vi "Get Algorithms.vi"(6 "Backend engine":T1, 8 "error in":errorcluster) -> (0 "error out":errorcluster, 3 "Available Algorithms":T2[](array[typedef]))   [LabVIEW 2013]
doc: "Get informations on all available Algorithms."
uses:
  TD Algorithm Information.ctl
  TD Backend Engine.ctl
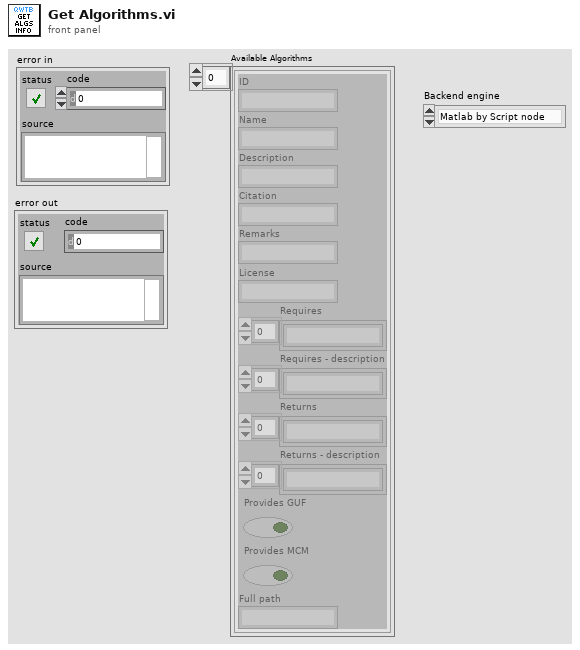
[diagram p1: front panel]
types:
  T1 = typedef "TD Backend Engine.ctl" = enum16{"Matlab by Script node", "GNU Octave by GOLPI"}
  T2 = typedef "TD Algorithm Information.ctl" = cluster{"ID":string, "Name":string, "Description":string, "Citation":string, "Remarks":string, "License":string, "Requires":string[], "Requires - description":string[], "Returns":string[], "Returns - description":string[], "Provides GUF":bool, "Provides MCM":bool, "Full path":string}
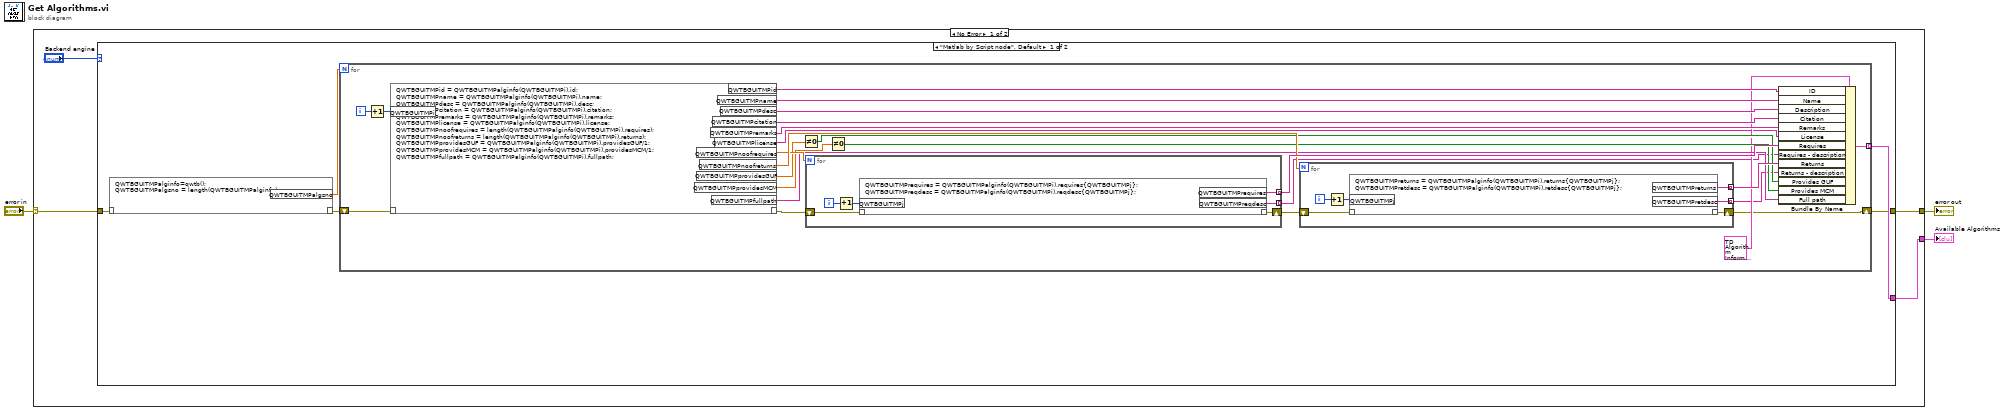
[diagram p0: block diagram]
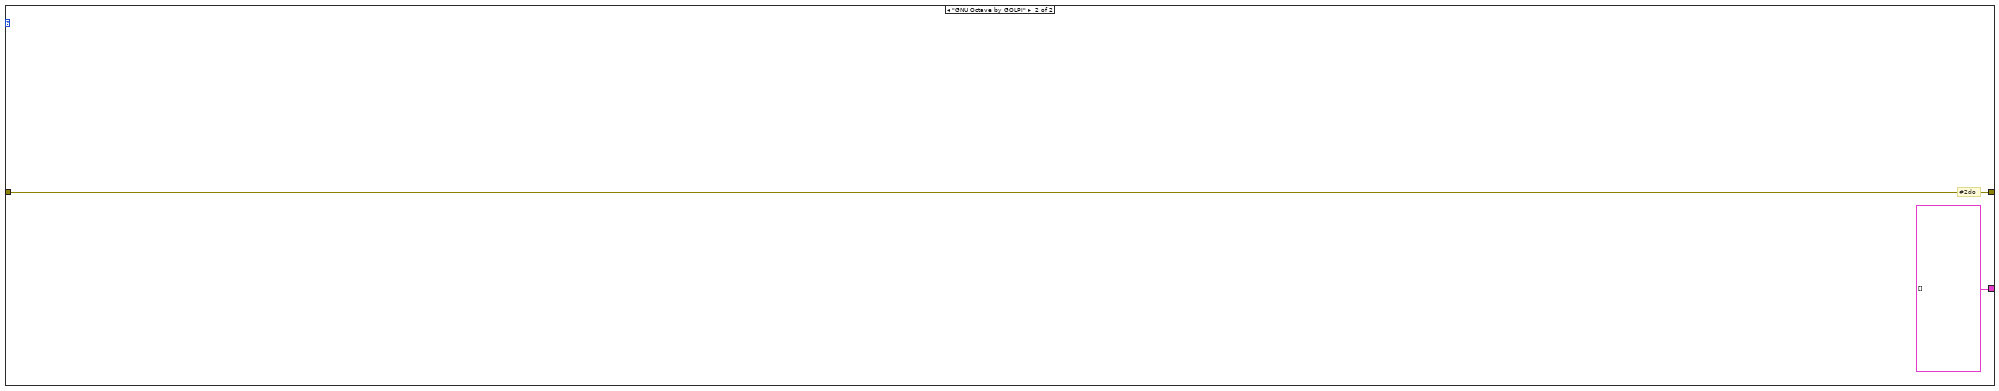
[diagram p2: hidden frame]
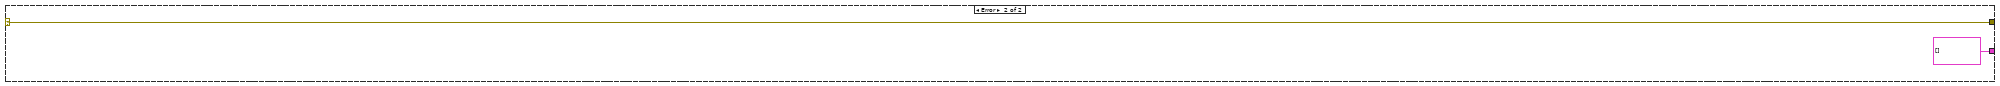
[diagram p3: hidden frame]
diagram:
  n1 = case shown="No Error" "error in" {
    selector: "error in" -> [w6 w53]
    tunnel: [w7 T2[] []] -> w3
    tunnel: [w5 w53] -> w1
    frame No Error {
      n2 = case shown="\"Matlab by Script node\", Default" "Backend engine" {
        tunnel: [w10 T2[] []] -> w7
        tunnel: w6 -> [w9 w51]
        tunnel: [w8 w51] -> w5
        frame "Matlab by Script node", Default {
          n3 = script code="QWTBGUITMPalginfo=qwtb();\nQWTBGUITMPalgsno = length(QWTBGUITMPalginfo);"("??"=w9) -> ("??"=w11:errorcluster, "QWTBGUITMPalgsno"=w12:dbl)
          n4 = for {
            N: w12 -> [_]
            tunnel: [w18] -> w10 mode=indexing
            shift-right: [w19] -> w8
            shift-left: w11 -> [w13]
            i -> [w37]
            n5 = Increment(x=w37) -> (x+1=w17:i32)
            n6 = script code="QWTBGUITMPid = QWTBGUITMPalginfo(QWTBGUITMPi).id;\nQWTBGUITMPname = QWTBGUITMPalginfo(QWTBGUITMPi).name;\nQWTBGUITMPdesc = QWTBGUITMPalginfo(QWTBGUITMPi).desc;\nQWTBGUITMPcitation = QWTBGUITMPalginfo(QWTBGUITMPi).citation;\nQWTBGUITMPremarks = QWTBGUITMPalginfo(QWTBGUITMPi).remarks;\nQWTBGUITMPlicense = QWTBGUITMPalginfo(QWTBGUITMPi).license;\nQWTBGUITMPnoofrequires = length(QWTBGUITMPalginfo(QWTBGUITMPi).requires);\nQWTBGUITMPnoofreturns = length(QWTBGUITMPalginfo(QWTBGUITMPi).returns);\nQWTBGUITMPprovidesGUF = QWTBGUITMPalginfo(QWTBGUITMPi).providesGUF/1;\nQWTBGUITMPprovidesMCM = QWTBGUITMPalginfo(QWTBGUITMPi).providesMCM/1;\nQWTBGUITMPfullpath = QWTBGUITMPalginfo(QWTBGUITMPi).fullpath;"("??"=w13, "QWTBGUITMPi"=w17) -> ("??"=w31:errorcluster, "QWTBGUITMPid"=w21:string, "QWTBGUITMPname"=w22:string, "QWTBGUITMPdesc"=w23:string, "QWTBGUITMPfullpath"=w24:string, "QWTBGUITMPnoofrequires"=w32:dbl, "QWTBGUITMPnoofreturns"=w34:dbl, "QWTBGUITMPcitation"=w30:string, "QWTBGUITMPremarks"=w29:string, "QWTBGUITMPprovidesGUF"=w27:dbl, "QWTBGUITMPprovidesMCM"=w25:dbl, "QWTBGUITMPlicense"=w14:string)
            n7 = Not Equal To 0?(x=w27) -> (x != 0?=w28:bool)
            n8 = for {
              N: w32 -> [_]
              shift-right: [w46] -> w33
              shift-left: w31 -> [w49]
              tunnel: [w45] -> w35 mode=indexing
              tunnel: [w44] -> w16 mode=indexing
              i -> [w47]
              n9 = Increment(x=w47) -> (x+1=w48:i32)
              n10 = script code="QWTBGUITMPrequires = QWTBGUITMPalginfo(QWTBGUITMPi).requires{QWTBGUITMPj};\nQWTBGUITMPreqdesc = QWTBGUITMPalginfo(QWTBGUITMPi).reqdesc{QWTBGUITMPj};"("??"=w49, "QWTBGUITMPj"=w48) -> ("??"=w46:errorcluster, "QWTBGUITMPrequires"=w45:string, "QWTBGUITMPreqdesc"=w44:string)
            }
            n11 = Not Equal To 0?(x=w25) -> (x != 0?=w26:bool)
            n12 = for {
              N: w34 -> [_]
              shift-right: [w40] -> w19
              shift-left: w33 -> [w43]
              tunnel: [w39] -> w36 mode=indexing
              tunnel: [w38] -> w15 mode=indexing
              i -> [w41]
              n13 = Increment(x=w41) -> (x+1=w42:i32)
              n14 = script code="QWTBGUITMPreturns = QWTBGUITMPalginfo(QWTBGUITMPi).returns{QWTBGUITMPj};\nQWTBGUITMPretdesc = QWTBGUITMPalginfo(QWTBGUITMPi).retdesc{QWTBGUITMPj};"("??"=w43, "QWTBGUITMPj"=w42) -> ("??"=w40:errorcluster, "QWTBGUITMPreturns"=w39:string, "QWTBGUITMPretdesc"=w38:string)
            }
            n15 = Bundle By Name(cluster=T2 {"ID"="", "Name"="", "Description"="", "Citation"="", "Remarks"="", "License"="", "Requires"=[], "Requires - description"=[], "Returns"=[], "Returns - description"=[], "Provides GUF"=FALSE, "Provides MCM"=FALSE, "Full path"=""} ("Algorithm Information"), "ID"=w21, "Name"=w22, "Description"=w23, "Citation"=w30, "Remarks"=w29, "License"=w14, "Requires"=w35, "Requires - description"=w16, "Returns"=w36, "Returns - description"=w15, "Provides GUF"=w28, "Provides MCM"=w26, "Full path"=w24) -> (w18:T2)
          }
        }
        frame "GNU Octave by GOLPI" {
          # "#2do"
        }
      }
    }
    frame Error {
    }
  }
  "Available Algorithms" <- w3
  "error out" <- w1
